vi "manual_update_last_id_ajuste_previo.vi"(8 "error in (no error)":errorcluster) -> (0 "error out":errorcluster, 3 "last_id_ajuste_previo":i32)   [LabVIEW 2019, in "Base de Datos.lvclass"]
uses:
  Base de Datos.lvclass
  Globals/globales.vi
panel:
  in  "last_id_ajuste_previo (manual)":i32
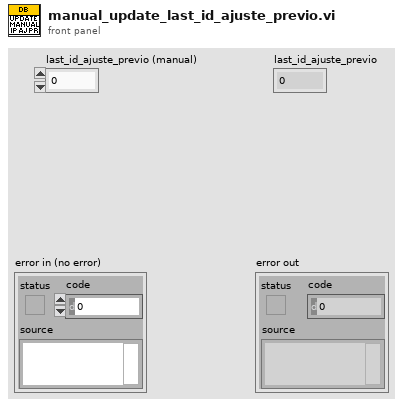
[diagram p1: front panel]
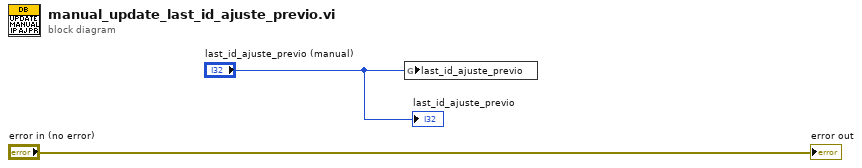
[diagram p0: block diagram]
diagram:
  n1 = global write "globales.vi" "last_id_ajuste_previo"("last_id_ajuste_previo (manual)") -> ()
  "error out" <- "error in (no error)"
  "last_id_ajuste_previo" <- "last_id_ajuste_previo (manual)"
